vi "File_SetLLBAsDir.vi"(1 "File names":string[](array[string]), 3 "Directory names":string[](array[string]), 5 "error in (no error)":errorcluster) -> (15 "File names out":string[](array[string]), 17 "Directory names out":string[](array[string]), 19 "error out":errorcluster)   [LabVIEW 2020]
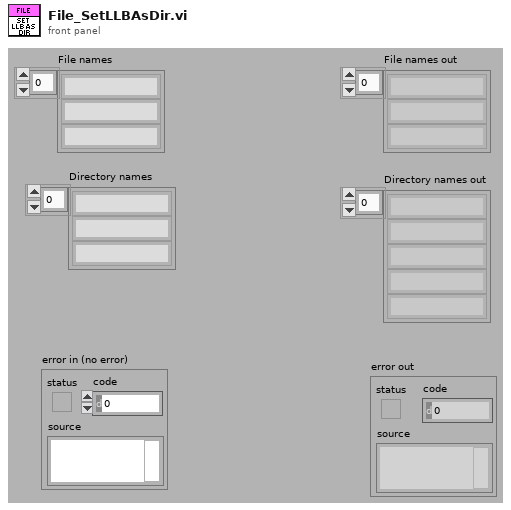
[diagram p1: front panel]
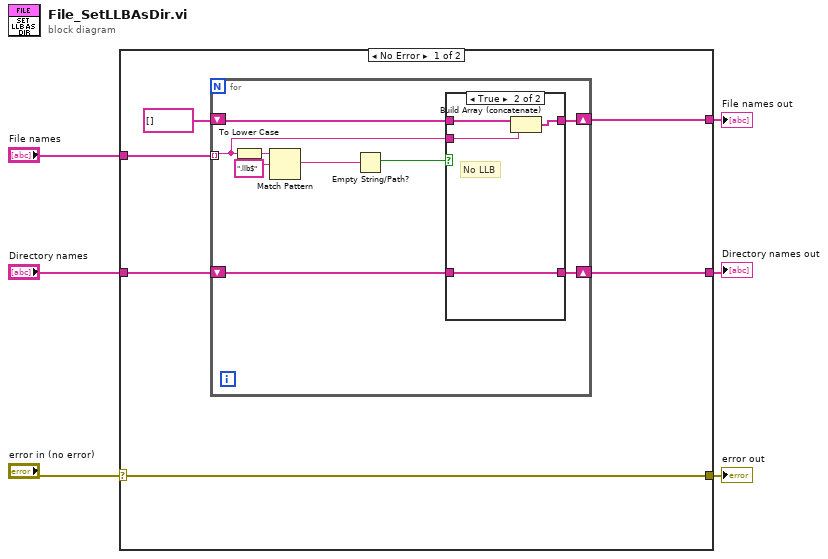
[diagram p0: block diagram]
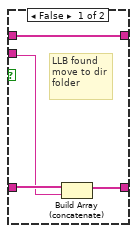
[diagram p2: hidden frame]
diagram:
  n1 = case shown="No Error" "error in (no error)" {
    selector: "error in (no error)" -> [w7 w32]
    tunnel: [w7 w32] -> w5
    tunnel: "File names" -> [w12 w31]
    tunnel: "Directory names" -> [w11 w30]
    tunnel: [w9 w31] -> w2
    tunnel: [w8 w30] -> w1
    frame No Error {
      n2 = for {
        tunnel: w12 -> [w18] mode=indexing
        shift-right: [w13] -> w8
        shift-left: w11 -> [w14]
        shift-right: [w17] -> w9
        shift-left: string[] [] ("File names") -> [w16]
        n3 = To Lower Case(string=w18) -> (all lower case string=w21:string)
        n4 = Match Pattern(string=w21, regular expression=".llb$") -> (match substring=w19:string)  [unwired: 4 out]
        n5 = Empty String/Path?(string/path=w19) -> (empty?=w15:bool)
        n6 = case shown="True" w15 {
          tunnel: w18 -> [w22 w27]
          tunnel: [w25 w29] -> w17
          tunnel: w16 -> [w25 w28]
          tunnel: w14 -> [w24 w26]
          tunnel: [w23 w26] -> w13
          frame False {
            # "LLB found\nmove to dir\nfolder"
            n7 = Build Array (concatenate)(w24, w22) -> (w23:string[])
          }
          frame True {
            # "No LLB"
            n8 = Build Array (concatenate)(w28, w27) -> (w29:string[])
          }
        }
      }
    }
    frame Error {
    }
  }
  "File names out" <- w2
  "Directory names out" <- w1
  "error out" <- w5
